vi "embeddingmodel_polymorphic.vi"   [LabVIEW 2020]
uses:
  llm_openai_embedding/llm_openai_embedding.lvclass
  llm_ollama_embedding/llm_ollama_embedding.lvclass
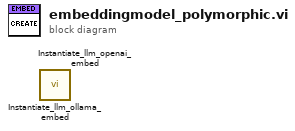
[diagram p0: block diagram]
diagram:
  n1 = call "Instantiate_llm_ollama_embed.vi"() -> ()  [unwired: 14 in, 2 out]
  n2 = call "Instantiate_llm_openai_embed.vi"() -> ()  [unwired: 14 in, 2 out]
